vi "主页面.vi"   [LabVIEW 2020]
panel:
  # "性能试验台"
types:
  T1 = enum32{"Invalid", "Standard", "Closed", "Hidden", "Minimized", "Maximized"}
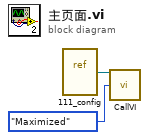
[diagram p0: block diagram]
diagram:
  n1 = vi-ref "111_config.vi"() -> (w2:refnum<vi>)
  n2 = call "CallVI.vi"("VI引用"=w2, "状态"=T1."Maximized") -> ()  [unwired: 11 in, 3 out]
